vi "ALTS-2015 LV2GBL Task Pass Fail Status.vi"(6 "States":T1=enum."Get", 8 "error in (no error)":errorcluster, 10 "Fail":bool=TRUE, 11 "Pass":bool=TRUE) -> (0 "error out":errorcluster, 2 "Fail Out":bool, 3 "Pass Out":bool)   [LabVIEW 2013]
uses:
  Controls/ALTS-2015 Pass Fail State.ctl
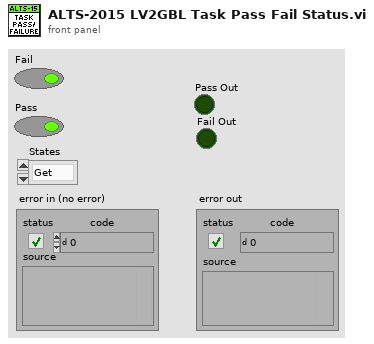
[diagram p1: front panel]
types:
  T1 = typedef "ALTS-2015 Pass Fail State.ctl" = enum16{"Set", "Get"}
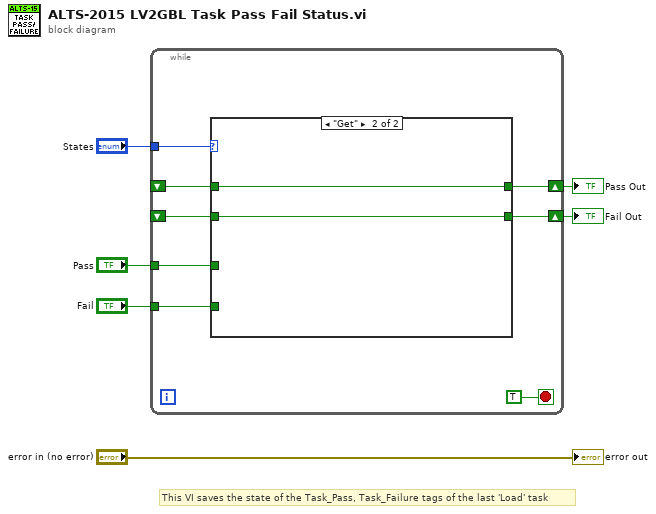
[diagram p0: block diagram]
diagram:
  # "This VI saves the state of the Task_Pass, Task_Failure tags of the last 'Load' task"
  n1 = while {
    tunnel: "States" -> [w14]
    shift-right: [w13] -> w4
    shift-left: _ -> [w11]
    tunnel: "Pass" -> [w12]
    shift-right: [w9] -> w2
    shift-left: _ -> [w8]
    tunnel: "Fail" -> [w10]
    stop <- TRUE stop-if-true
    n2 = case shown="\"Get\"" w14 {
      tunnel: [w16 w18] -> w13
      tunnel: w12 -> [w16 _]
      tunnel: w11 -> [_ w18]
      tunnel: w10 -> [w15 _]
      tunnel: [w15 w17] -> w9
      tunnel: w8 -> [_ w17]
      frame "Set", Default {
      }
      frame "Get" {
      }
    }
  }
  "Pass Out" <- w4
  "Fail Out" <- w2
  "error out" <- "error in (no error)"
